vi "ACQ encoders read values.vi"(8 "error in (no error)":errorcluster, 11 "Tasks ref in":T1) -> (0 "error out":errorcluster, 2 "Encoders out":dbl[](array[numeric]), 3 "Tasks ref out":T1)   [LabVIEW 2013]
doc: "Use this template to build a VI to use as a subVI."
uses:
  Kontrolki/KartaDAQ/ACQ all read tasks.ctl
  <vilib>/DAQmx/read.llb/DAQmx Read.vi
  <vilib>/DAQmx/read.llb/DAQmx Read (Counter DBL 1Chan 1Samp).vi
  <vilib>/DAQmx/miscellaneous.llb/DAQmx Fill In Error Info.vi
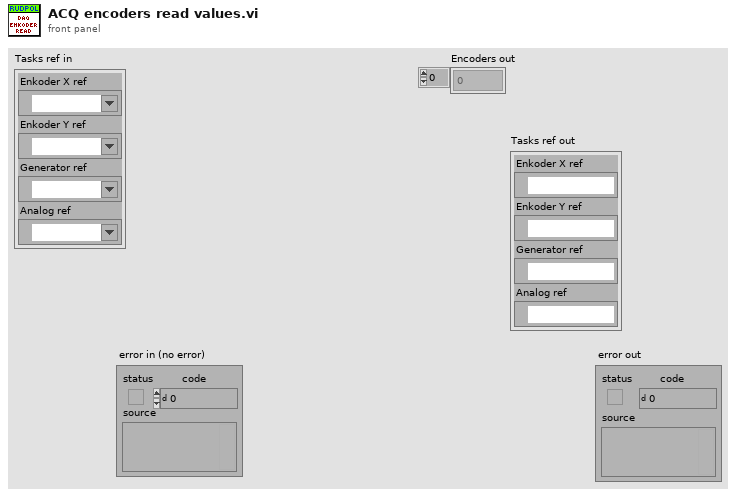
[diagram p1: front panel]
types:
  T1 = typedef "ACQ all read tasks.ctl" = cluster{"Enkoder X ref":refnum<k21>, "Enkoder Y ref":refnum<k21>, "Generator ref":refnum<k21>, "Analog ref":refnum<k21>}
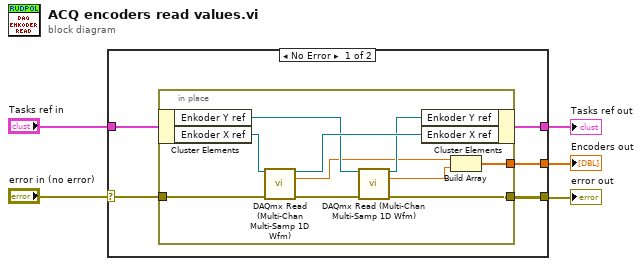
[diagram p0: block diagram]
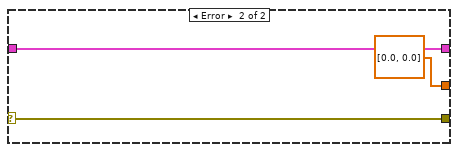
[diagram p2: hidden frame]
diagram:
  n1 = case shown="No Error" "error in (no error)" {
    selector: "error in (no error)" -> [w9 w23]
    tunnel: [w8 w23] -> w4
    tunnel: "Tasks ref in" -> [w10 w22]
    tunnel: [w6 w22] -> w1
    tunnel: [w7 dbl[] [0.0, 0.0]] -> w3
    frame No Error {
      n2 = in-place {
        in-place-border: w9 -> [w19]
        in-place-border: [w18] -> w8
        in-place-border: [w11] -> w7
        n3 = in-place-cluster #1(w10) -> ("Enkoder Y ref"=w15:refnum<k21>, "Enkoder X ref"=w17:refnum<k21>)
        n4 = call-poly "DAQmx Read (Multi-Chan Multi-Samp 1D Wfm).vi"("task/channels in"=w17, "error in"=w19) -> ("task out"=w16:refnum<k21>, "data"=w12:dbl, "error out"=w20:errorcluster)  [unwired: 11 in]
        n5 = call-poly "DAQmx Read (Multi-Chan Multi-Samp 1D Wfm).vi"("task/channels in"=w15, "error in"=w20) -> ("task out"=w14:refnum<k21>, "data"=w13:dbl, "error out"=w18:errorcluster)  [unwired: 11 in]
        n6 = in-place-cluster #1("Enkoder Y ref"=w14, "Enkoder X ref"=w16) -> (w6:T1)
        n7 = Build Array(w12, w13) -> (w11:dbl[])
      }
    }
    frame Error {
    }
  }
  "error out" <- w4
  "Encoders out" <- w3
  "Tasks ref out" <- w1
